vi "MaskFilters.vi"(6 "ImgY":i32, 7 "FilterParam":cluster{"D0":u16, "D1":u16, "u0":i16, "v0":i16}={"D0"=0, "D1"=0, "u0"=10, "v0"=30}, 8 "EorIn":errorcluster, 9 "ImgX":i32, 11 "Filter":T1(ring)) -> (0 "ErrOut":errorcluster, 1 "H(u,v)":u8[][](array[numeric]))   [LabVIEW 2014]
doc: "Use this template to build a VI to use as a subVI."
panel:
  # "Output Parameters"
  # "Input Parameters"
  # "1) low/high pass filter controlled by D0;\n2) Band pass/reject controlled by D0(low cut) and D1(high cut);\n3) Notch Filter controlled by (+/-u0,+/-v0) and D0;"
  # "VI Description:\nThis VI is .."
  # ":: MVi Framework V1.0 ::\nAuthor:Gaoke Yang\nEmail: gaoke.yang@yahoo.com\nWeb: www.mvicontrol.com\nCopyright (C) 2015, MVI Technologies All Rights Reserved"
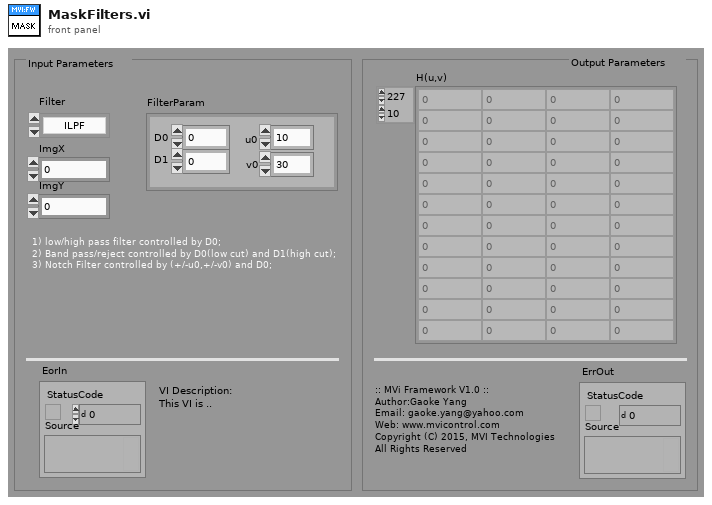
[diagram p1: front panel]
types:
  T1 = enum16{"ILPF", "IHPF", "IBPF", "IBRF", "INPF", "INRF"}
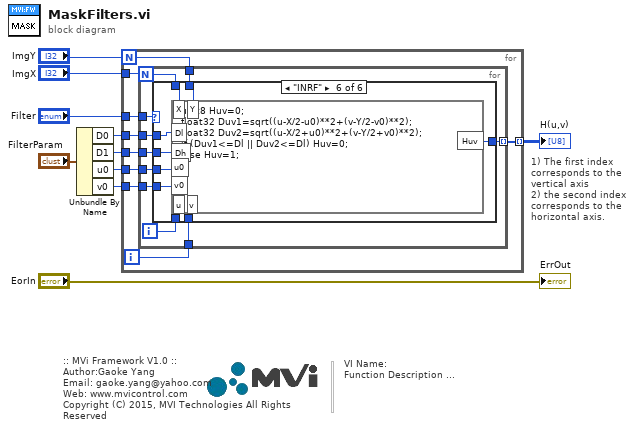
[diagram p0: block diagram]
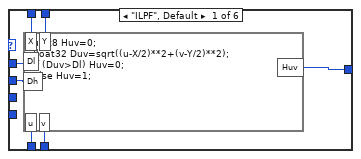
[diagram p2: hidden frame]
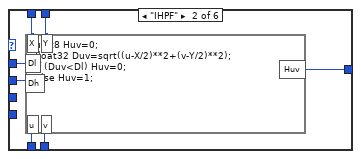
[diagram p3: hidden frame]
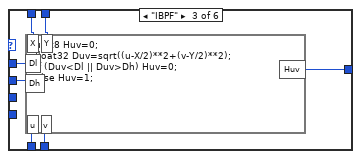
[diagram p4: hidden frame]
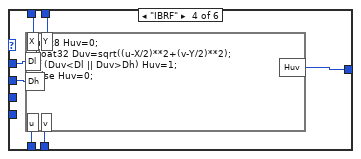
[diagram p5: hidden frame]
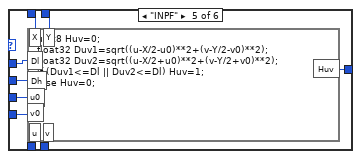
[diagram p6: hidden frame]
diagram:
  # "1) The first index corresponds to the vertical axis \n2) the second index corresponds to the horizontal axis."
  # "VI Name:\nFunction Description ..."
  # ":: MVi Framework V1.0 ::\nAuthor:Gaoke Yang\nEmail: gaoke.yang@yahoo.com\nWeb: www.mvicontrol.com\nCopyright (C) 2015, MVI Technologies All Rights Reserved"
  n1 = Unbundle By Name("FilterParam") -> ("D0"=w4:u16, "D1"=w3:u16, "u0"=w2:i16, "v0"=w1:i16)
  n2 = for {
    N: "ImgY" -> [w13]
    tunnel: "ImgX" -> [w19]
    tunnel: "Filter" -> [w18]
    tunnel: w4 -> [w17]
    tunnel: w3 -> [w16]
    tunnel: w2 -> [w15]
    tunnel: [w12] -> w6 mode=indexing
    tunnel: w1 -> [w11]
    i -> [w14]
    n3 = for {
      N: w19 -> [w23]
      tunnel: w18 -> [w29]
      tunnel: w17 -> [w28]
      tunnel: w16 -> [w27]
      tunnel: w15 -> [w26]
      tunnel: w14 -> [w24]
      tunnel: w13 -> [w22]
      tunnel: [w21] -> w12 mode=indexing
      tunnel: w11 -> [w20]
      i -> [w25]
      n4 = case shown="\"INRF\"" w29 {
        tunnel: w28 -> [w32 w39 w47 w51 w60 w69]
        tunnel: w27 -> [w33 w40 w46 w52 w61 w70]
        tunnel: w26 -> [_ _ _ _ w59 w68]
        tunnel: w25 -> [w35 w41 w45 w54 w63 w72]
        tunnel: w24 -> [w34 w42 w44 w53 w62 w71]
        tunnel: w23 -> [w31 w38 w49 w56 w65 w74]
        tunnel: w22 -> [w30 w37 w48 w55 w64 w73]
        tunnel: [w36 w43 w50 w57 w66 w75] -> w21
        tunnel: w20 -> [_ _ _ _ w58 w67]
        frame "ILPF", Default {
          n5 = formula code="uInt8 Huv=0;\nfloat32 Duv=sqrt((u-X/2)**2+(v-Y/2)**2);\nif (Duv>Dl) Huv=0;\nelse Huv=1;"("u"=w35, "v"=w34, "Dl"=w32, "Y"=w30, "X"=w31, "Dh"=w33) -> ("Huv"=w36:u8)
        }
        frame "IHPF" {
          n6 = formula code="uInt8 Huv=0;\nfloat32 Duv=sqrt((u-X/2)**2+(v-Y/2)**2);\nif (Duv<Dl) Huv=0;\nelse Huv=1;"("u"=w41, "v"=w42, "Dl"=w39, "Y"=w37, "X"=w38, "Dh"=w40) -> ("Huv"=w43:u8)
        }
        frame "IBPF" {
          n7 = formula code="uInt8 Huv=0;\nfloat32 Duv=sqrt((u-X/2)**2+(v-Y/2)**2);\nif (Duv<Dl || Duv>Dh) Huv=0;\nelse Huv=1;"("u"=w45, "v"=w44, "Dl"=w47, "Y"=w48, "X"=w49, "Dh"=w46) -> ("Huv"=w50:u8)
        }
        frame "IBRF" {
          n8 = formula code="uInt8 Huv=0;\nfloat32 Duv=sqrt((u-X/2)**2+(v-Y/2)**2);\nif (Duv<Dl || Duv>Dh) Huv=1;\nelse Huv=0;"("u"=w54, "v"=w53, "Dl"=w51, "Y"=w55, "X"=w56, "Dh"=w52) -> ("Huv"=w57:u8)
        }
        frame "INPF" {
          n9 = formula code="uInt8 Huv=0;\nfloat32 Duv1=sqrt((u-X/2-u0)**2+(v-Y/2-v0)**2);\nfloat32 Duv2=sqrt((u-X/2+u0)**2+(v-Y/2+v0)**2);\nif (Duv1<=Dl || Duv2<=Dl) Huv=1;\nelse Huv=0;"("u"=w63, "v"=w62, "Dl"=w60, "Y"=w64, "X"=w65, "Dh"=w61, "u0"=w59, "v0"=w58) -> ("Huv"=w66:u8)
        }
        frame "INRF" {
          n10 = formula code="uInt8 Huv=0;\nfloat32 Duv1=sqrt((u-X/2-u0)**2+(v-Y/2-v0)**2);\nfloat32 Duv2=sqrt((u-X/2+u0)**2+(v-Y/2+v0)**2);\nif (Duv1<=Dl || Duv2<=Dl) Huv=0;\nelse Huv=1;"("u"=w72, "v"=w71, "Dl"=w69, "Y"=w73, "X"=w74, "Dh"=w70, "u0"=w68, "v0"=w67) -> ("Huv"=w75:u8)
        }
      }
    }
  }
  "H(u,v)" <- w6
  "ErrOut" <- "EorIn"
